vi "Stop AsyncSum.vi"(8 "error in (no error)":errorcluster, 9 "LVUserEventCallBackRef":refnum<user-event>, 10 "Handle":u64, 11 "path in":path) -> (0 "error out":errorcluster, 3 "dup path":path)   [LabVIEW 2016, in "DemoSkeleton.lvlib"]
uses:
  DemoSkeleton.lvlib
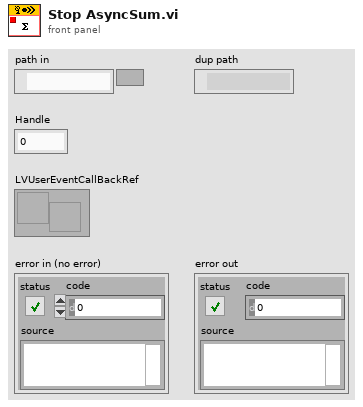
[diagram p1: front panel]
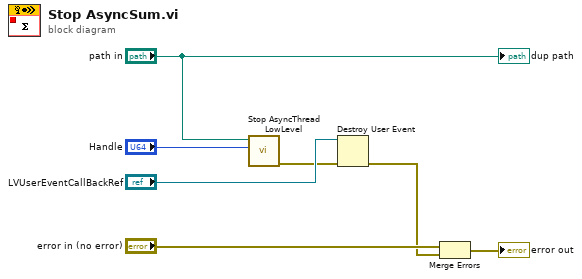
[diagram p0: block diagram]
diagram:
  n1 = call "Stop AsyncThread LowLevel.vi"("Handle"="Handle", "path in"="path in") -> ("error out"=w2:errorcluster)  [unwired: 8 in, 1 out]
  n2 = Destroy User Event(user event="LVUserEventCallBackRef", error in=w2) -> (error out=w1:errorcluster)
  n3 = Merge Errors("error in (no error)", w1) -> (→"error out":errorcluster)
  "dup path" <- "path in"
